vi "RefnumToNum.vi"(1 "Refnum in":refnum<k20>) -> (0 "Reference ID":u64)   [LabVIEW 2023]
doc: "Converts FPGA refnum to numeric reference ID"
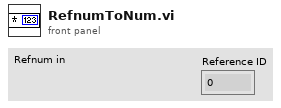
[diagram p1: front panel]
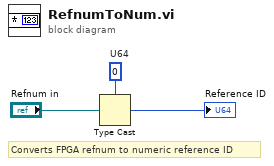
[diagram p0: block diagram]
diagram:
  w2 = u64 0  # U64
  # "Converts FPGA refnum to numeric reference ID"
  n1 = Type Cast(type=w2, x="Refnum in") -> (*(type *) &x=→"Reference ID":u64)
